vi "Istwert abholen.vi"(7 "automatisch":bool, 8 "error in (no error)":errorcluster caption="Fehler (Eingang, kein Fehler)", 9 "Position Index in":i32, 10 "Eingangswerte":T1, 11 "Gasindex":i32) -> (0 "error out":errorcluster caption="Fehler (Ausgang)", 1 "Position Index out":i32)   [LabVIEW 2020, in "Linearisierung v2.lvlib"]
uses:
  Linearisierung v2.lvlib
  Aktion Lin Daten aufarbeiten.ctl
  Allgemein/allgemeine Sub-VIs.lvlib
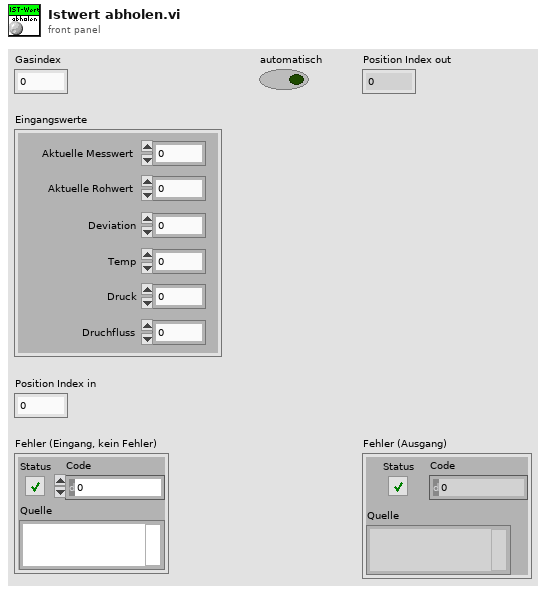
[diagram p1: front panel]
types:
  T1 = cluster{"Aktuelle Messwert":dbl, "Aktuelle Rohwert":dbl, "Deviation":dbl, "Temp":dbl, "Druck":dbl, "Druchfluss":dbl}
  T2 = typedef "Linearisierung v2.lvlib/Aktion Lin Daten aufarbeiten.ctl" = enum16{"lesen", "Protkolldaten", "speichern", "laden", "EPA auswerten", "Tabelle schreiben", "Lin auswerten", "Tab init", "Stufentabelle", "EPA aktiviert", "Nachbehandlung laden", "Tabelle löschen", "Istwerte löschen", "Zeile löschen", "Zeile einfügen", "LIN aktiviert", "LIN/EPA aktiv laden", "EGAK Tab", "LIN übernehmen", "Tab init ohne Stufen"}
  T3 = typedef "Linearisierung v2.lvlib/Eingabetabelle.ctl" = string[][]
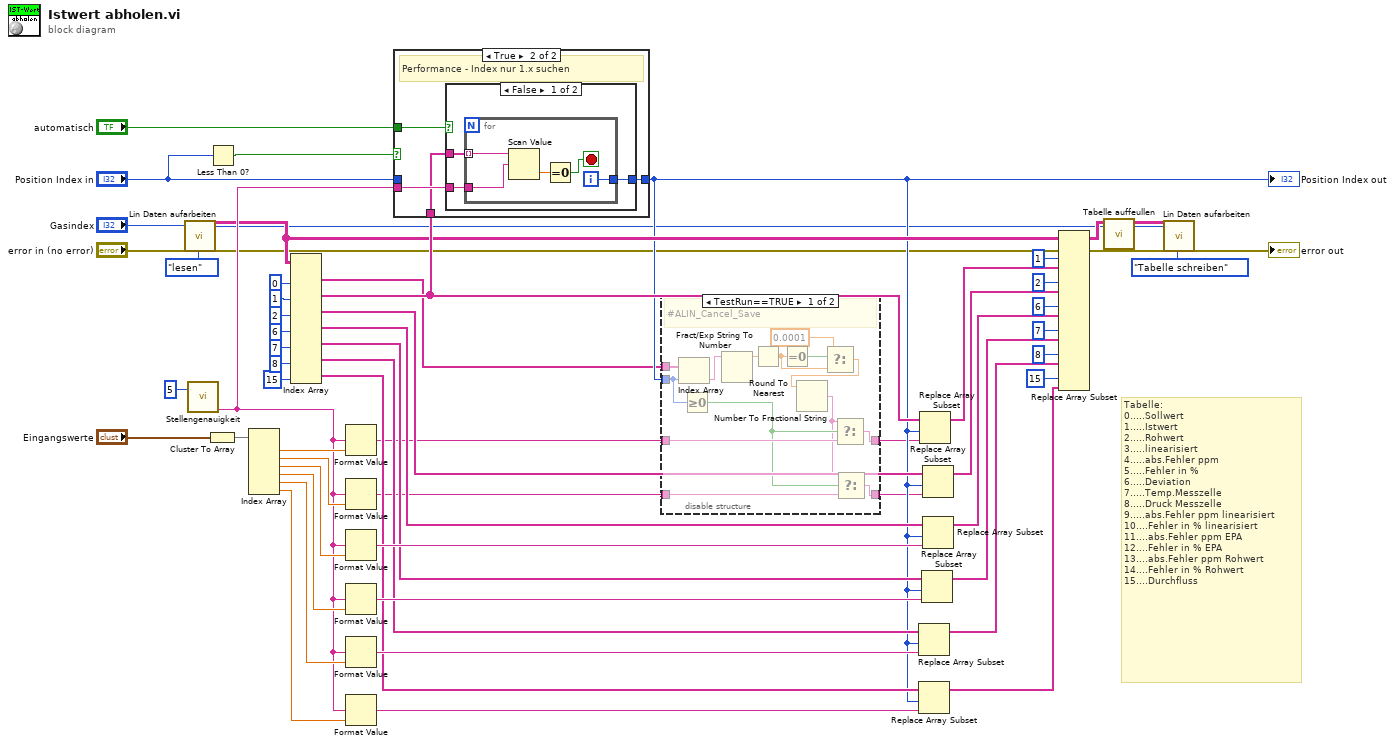
[diagram p0: block diagram]
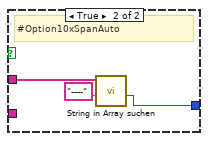
[diagram p3: hidden frame]
diagram:
  # "Tabelle:\n0.....Sollwert\n1.....Istwert\n2.....Rohwert\n3.....linearisiert\n4.....abs.Fehler ppm\n5.....Fehler in %\n6.....Deviation\n7.....Temp.Messzelle\n8.....Druck Messzelle\n9.....abs.Fehler ppm linearisiert\n10....Fehler in % linearisiert\n11....abs.Fehler ppm EPA\n12....Fehler in % EPA\n13....abs.Fehler ppm Rohwert\n14....Fehler in % Rohwert\n15....Durchfluss"
  n1 = call "Lin Daten aufarbeiten.vi"("Index (Seite)"="Gasindex", "error in (no error)"="error in (no error)", "Aktionen"=Aktion_Lin_Daten_aufarbeiten."lesen") -> ("Eingabetabelle"=w13:T3, "Index (Seite) out"=w3:i32, "error out"=w5:errorcluster)  [unwired: 14 in, 8 out]
  n2 = call "Stellengenauigkeit.vi"("Genauigkeit (6)"=i16 5) -> ("Formatstring"=w24:string)  [unwired: 9 in, 1 out]
  n3 = Cluster To Array(cluster="Eingangswerte") -> (array=w50:dbl[])
  n4 = Less Than 0?(x="Position Index in") -> (x < 0?=w7:bool)
  n5 = Index Array(array=w50) -> (element #1=w49:dbl, element #2=w48:dbl, element #3=w47:dbl, element #4=w46:dbl, element #5=w45:dbl, element #6=w19:dbl)  [unwired: 6 in]
  n6 = Index Array(array=w13, index (col) #1=0 ("Deaktivierter Index (Spalte)"), index (col) #2=1 ("Deaktivierter Index (Spalte)"), index (col) #3=2 ("Index (Spalte)"), index (col) #4=6 ("Index (Spalte)"), index (col) #5=7 ("Index (Spalte)"), index (col) #6=8 ("Index (Spalte)"), index (col) #7=15 ("Index (Spalte)")) -> (element #1=w10:string[], element #2=w17:string[], element #3=w16:string[], element #4=w35:string[], element #5=w34:string[], element #6=w33:string[], element #7=w22:string[])  [unwired: 7 in]
  n7 = Format Value(format string=w24, value (0)=w49) -> (output string=w9:string)  [unwired: 1 in]
  n8 = Format Value(format string=w24, value (0)=w48) -> (output string=w2:string)  [unwired: 1 in]
  n9 = Format Value(format string=w24, value (0)=w47) -> (output string=w38:string)  [unwired: 1 in]
  n10 = Format Value(format string=w24, value (0)=w46) -> (output string=w37:string)  [unwired: 1 in]
  n11 = Format Value(format string=w24, value (0)=w45) -> (output string=w36:string)  [unwired: 1 in]
  n12 = Format Value(format string=w24, value (0)=w19) -> (output string=w25:string)  [unwired: 1 in]
  n13 = case shown="True" w7 {
    tunnel: w24 -> [_ w63]
    tunnel: "automatisch" -> [_ w62]
    tunnel: w17 -> [_ w61]
    tunnel: [w59 w60] -> w12
    tunnel: "Position Index in" -> [w59 _]
    frame False {
    }
    frame True {
      # "Performance - Index nur 1.x suchen"
      n14 = case shown="False" w62 {
        tunnel: w61 -> [w66 w73]
        tunnel: w63 -> [w65 _]
        tunnel: [w64 w72] -> w60
        frame False {
          n15 = for {
            tunnel: w66 -> [w70] mode=indexing
            tunnel: w65 -> [w71]
            tunnel: [w67] -> w64
            i -> [w67]
            stop <- w68 stop-if-true
            n16 = Scan Value(string=w70, format string=w71) -> (value=w69:dbl)  [unwired: 1 in, 1 out]
            n17 = Equal To 0?(x=w69) -> (x = 0?=w68:bool)
          }
        }
        frame True {
          # "#Option10xSpanAuto"
          n18 = call "String in Array suchen.vi"("Nach String/Zeichen suchen (-)"="----", "String-Array"=w73) -> ("Index"=w72:i32)  [unwired: 7 in, 2 out]
        }
      }
    }
  }
  "Position Index out" <- w12
  n19 = disable-structure shown="TestRun==TRUE" {
    disable-tunnel: w10 -> [w84 _]
    disable-tunnel: w9 -> [w87 w90]
    disable-tunnel: [w88 w90] -> w8
    disable-tunnel: w12 -> [w83 _]
    disable-tunnel: w2 -> [w78 w89]
    disable-tunnel: [w76 w89] -> w1
    frame condition #0 {
      # "#ALIN_Cancel_Save"
      n20 = Index Array(array=w84, index=w83) -> (element=w85:string)
      n21 = Greater Or Equal To 0?(x=w83) -> (x >= 0?=w77:bool)
      n22 = Fract/Exp String To Number(string=w85) -> (number=w86:dbl)  [unwired: 3 in, 1 out]
      n23 = Round To Nearest(number=w86) -> (nearest integer value=w81:dbl)
      n24 = Equal To 0?(x=w81) -> (x = 0?=w82:bool)
      n25 = Select(t=0.0001, s=w82, f=w81) -> (s? t:f=w79:dbl)
      n26 = Number To Fractional String(number=w79) -> (F-format string=w75:string)  [unwired: 3 in]
      n27 = Select(t=w75, s=w77, f=w87) -> (s? t:f=w88:string)
      n28 = Select(t=w75, s=w77, f=w78) -> (s? t:f=w76:string)
    }
    frame condition #1 (active) {
    }
  }
  n29 = Replace Array Subset(array=w33, new element=w36, index=w12) -> (w30:string[])
  n30 = Replace Array Subset(array=w22, new element=w25, index=w12) -> (w20:string[])
  n31 = Replace Array Subset(array=w17, new element=w8, index=w12) -> (w57:string[])
  n32 = Replace Array Subset(array=w34, new element=w37, index=w12) -> (w31:string[])
  n33 = Replace Array Subset(array=w16, new element=w1, index=w12) -> (w52:string[])
  n34 = Replace Array Subset(array=w35, new element=w38, index=w12) -> (w32:string[])
  n35 = Replace Array Subset(array=w13, new element #1=w57, index (col) #1=1 ("Deaktivierter Index (Spalte)"), new element #2=w52, index (col) #2=2 ("Index (Spalte)"), new element #3=w32, index (col) #3=6 ("Index (Spalte)"), new element #4=w31, index (col) #4=7 ("Index (Spalte)"), new element #5=w30, index (col) #5=8 ("Index (Spalte)"), new element #6=w20, index (col) #6=15 ("Index (Spalte)")) -> (w29:T3)  [unwired: 6 in]
  n36 = call "Tabelle auffeullen.vi"("Neue Tabelle"=w29) -> ("Tabelle"=w26:string[][])  [unwired: 10 in]
  n37 = call "Lin Daten aufarbeiten.vi"("Eingabetabelle"=w26, "Index (Seite)"=w3, "error in (no error)"=w5, "Aktionen"=Aktion_Lin_Daten_aufarbeiten."Tabelle schreiben") -> ("error out"=→"error out":errorcluster)  [unwired: 13 in, 10 out]
